vi "Sect02-Single File_Write Results.vi"(8 "error in (no error)":errorcluster, 11 "QSM_ShiftRegister_TEST in":T1 {"ROI Process"."Particle Variables" items=["Center of Mass X", "Center of Mass Y", "First Pixel X", "First Pixel Y", "Bounding Rect Left", "Bounding Rect Top", "Bounding Rect Right", "Bounding Rect Bottom", "Max Feret Diameter Start X", "Max Feret Diameter Start Y", "Max Feret Diameter End X", "Max Feret Diameter End Y", "Max Horiz. Segment Length Left", "Max Horiz. Segment Length Right", "Max Horiz. Segment Length Row", "-", "Bounding Rect Width", "Bounding Rect Height", "Bounding Rect Diagonal", "Perimeter", "Convex Hull Perimeter", "Holes' Perimeter", "Max Feret Diameter", "Equivalent Ellipse Major Axis", "Equivalent Ellipse Minor Axis", "Equivalent Ellipse Minor Axis (Feret)", "Equivalent Rect Long Side", "Equivalent Rect Short Side", "Equivalent Rect Diagonal", "Equivalent Rect Short Side (Feret)", "Average Horiz. Segment Length", "Average Vert. Segment Length", "Hydraulic Radius", "Waddel Disk Diameter", "-", "Area", "Holes' Area", "Particle & Holes' Area", "Convex Hull Area", "Image Area", "-", "Number of Holes", "Number of Horiz. Segments", "Number of Vert. Segments", "-", "Orientation", "Max Feret Diameter Orientation", "-", "% Area/Image Area", "% Area/(Particle & Holes' Area)", "Ratio of Equivalent Ellipse Axes", "Ratio of Equivalent Rect Sides", "-", "Elongation Factor", "Compactness Factor", "Heywood Circularity Factor", "Type Factor", "-", "Sum X", "Sum Y", "Sum XX", "Sum XY", "Sum YY", "Sum XXX", "Sum XXY", "Sum XYY", "Sum YYY", "-", "Moment of Inertia XX", "Moment of Inertia XY", "Moment of Inertia YY", "Moment of Inertia XXX", "Moment of Inertia XXY", "Moment of Inertia XYY", "Moment of Inertia YYY", "Norm. Moment of Inertia XX", "Norm. Moment of Inertia XY", "Norm. Moment of Inertia YY", "Norm. Moment of Inertia XXX", "Norm. Moment of Inertia XXY", "Norm. Moment of Inertia XYY", "Norm. Moment of Inertia YYY", "Hu Moment 1", "Hu Moment 2", "Hu Moment 3", "Hu Moment 4", "Hu Moment 5", "Hu Moment 6", "Hu Moment 7"]; "ROI Process"."Particle Measurements (Pixels)" format="%.2f"; "ROI Process"."ROIS"."Contours"."Type" items=["No Selection", "Point", "Line", "Rectangle", "Oval", "Polygon", "Freehand Region", "Annulus", "Unused2", "Unused3", "Broken Line", "Freehand Line", "Rotated Rectangle"]; "Single Image Results"."ROI Results"."LIMLOCALMETADATA"."dTimeMSec" format="%.2f"}) -> (0 "error out":errorcluster, 3 "QSM_ShiftRegister_TEST out":T1 {"ROI Process"."Particle Variables" items=["Center of Mass X", "Center of Mass Y", "First Pixel X", "First Pixel Y", "Bounding Rect Left", "Bounding Rect Top", "Bounding Rect Right", "Bounding Rect Bottom", "Max Feret Diameter Start X", "Max Feret Diameter Start Y", "Max Feret Diameter End X", "Max Feret Diameter End Y", "Max Horiz. Segment Length Left", "Max Horiz. Segment Length Right", "Max Horiz. Segment Length Row", "-", "Bounding Rect Width", "Bounding Rect Height", "Bounding Rect Diagonal", "Perimeter", "Convex Hull Perimeter", "Holes' Perimeter", "Max Feret Diameter", "Equivalent Ellipse Major Axis", "Equivalent Ellipse Minor Axis", "Equivalent Ellipse Minor Axis (Feret)", "Equivalent Rect Long Side", "Equivalent Rect Short Side", "Equivalent Rect Diagonal", "Equivalent Rect Short Side (Feret)", "Average Horiz. Segment Length", "Average Vert. Segment Length", "Hydraulic Radius", "Waddel Disk Diameter", "-", "Area", "Holes' Area", "Particle & Holes' Area", "Convex Hull Area", "Image Area", "-", "Number of Holes", "Number of Horiz. Segments", "Number of Vert. Segments", "-", "Orientation", "Max Feret Diameter Orientation", "-", "% Area/Image Area", "% Area/(Particle & Holes' Area)", "Ratio of Equivalent Ellipse Axes", "Ratio of Equivalent Rect Sides", "-", "Elongation Factor", "Compactness Factor", "Heywood Circularity Factor", "Type Factor", "-", "Sum X", "Sum Y", "Sum XX", "Sum XY", "Sum YY", "Sum XXX", "Sum XXY", "Sum XYY", "Sum YYY", "-", "Moment of Inertia XX", "Moment of Inertia XY", "Moment of Inertia YY", "Moment of Inertia XXX", "Moment of Inertia XXY", "Moment of Inertia XYY", "Moment of Inertia YYY", "Norm. Moment of Inertia XX", "Norm. Moment of Inertia XY", "Norm. Moment of Inertia YY", "Norm. Moment of Inertia XXX", "Norm. Moment of Inertia XXY", "Norm. Moment of Inertia XYY", "Norm. Moment of Inertia YYY", "Hu Moment 1", "Hu Moment 2", "Hu Moment 3", "Hu Moment 4", "Hu Moment 5", "Hu Moment 6", "Hu Moment 7"]; "ROI Process"."Particle Measurements (Pixels)" format="%.2f"; "ROI Process"."ROIS"."Contours"."Type" items=["No Selection", "Point", "Line", "Rectangle", "Oval", "Polygon", "Freehand Region", "Annulus", "Unused2", "Unused3", "Broken Line", "Freehand Line", "Rotated Rectangle"]; "Single Image Results"."ROI Results"."LIMLOCALMETADATA"."dTimeMSec" format="%.2f"})   [LabVIEW 2014, in "TestQSM.lvlib"]
uses:
  TestQSM.lvlib
  Controls/QSM_ShiftRegister.ctl
  QueueMaintenance/TypeDef/QSMRef_ALL.ctl
  Queue_TESTGUIUPDATE/Controls/QSM_Reference.ctl
  Queue_TESTGUIUPDATE/Controls/QSM_DataType.ctl
  Queue_TESTGUIUPDATE/Controls/QSM_RunStates.ctl
  Controls/QSM_Reference.ctl
  Controls/QSM_DataType.ctl
  Controls/QSM_RunStates.ctl
  Custom Controls/cluster - Image Results.ctl
  ND2_Reader_32bit/controls/cluster_LIMLOCALMETADATA.ctl
  FileIO/TypeDef - File Actions.ctl
  Queue_TESTGUIUPDATE/GUIUpdateQSM.lvlib
  QueueMaintenance/QueueMaintenance.lvlib
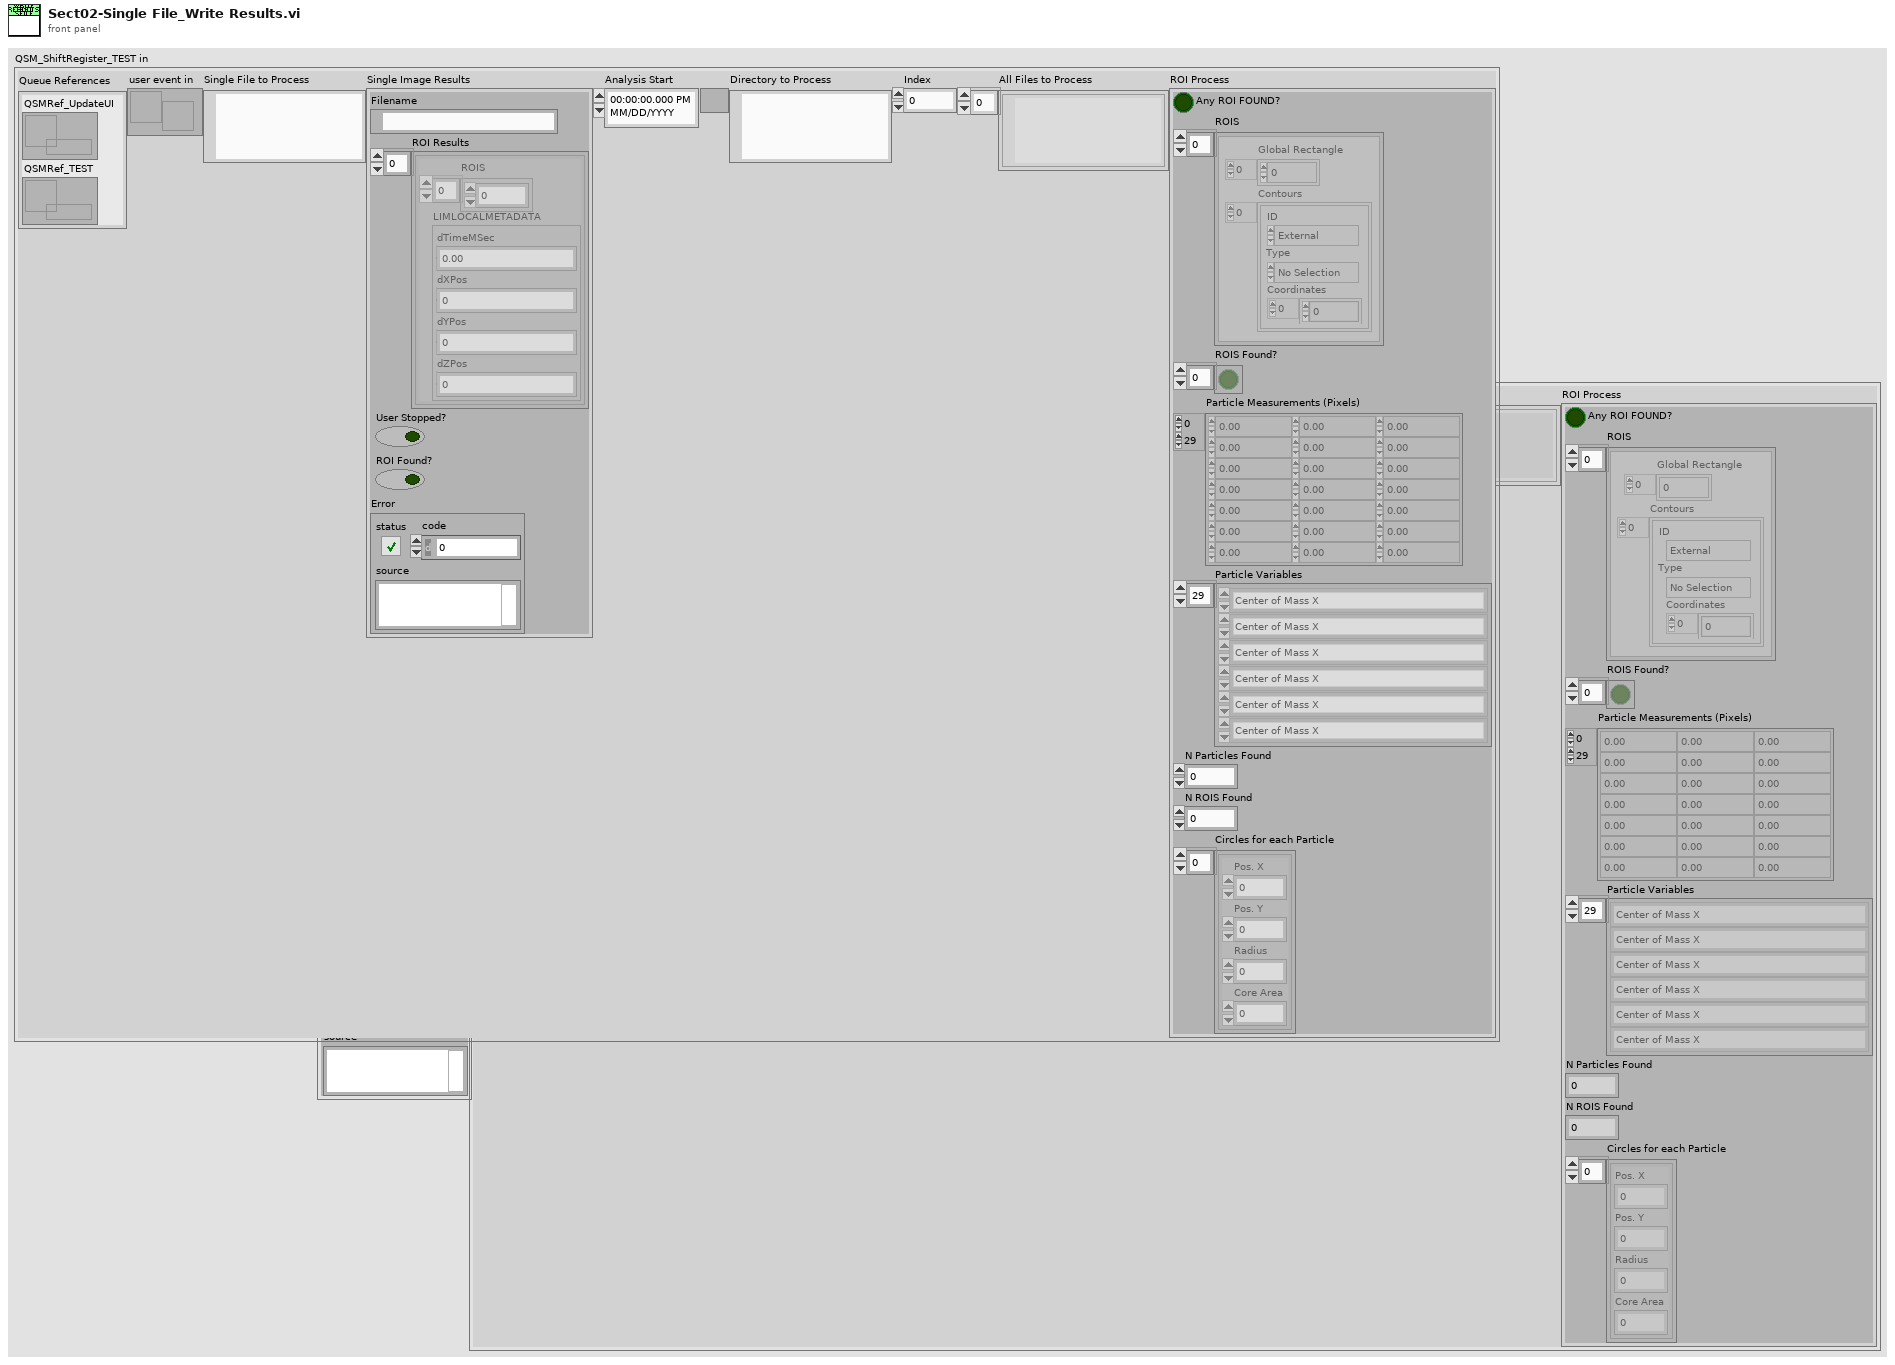
[diagram p1: front panel]
types:
  T1 = typedef "TestQSM.lvlib/QSM_ShiftRegister.ctl" = cluster{"Queue References":T2, "user event in":refnum<user-event>, "Single File to Process":path, "Single Image Results":T5, "Analysis Start":timestamp, "Directory to Process":path, "Index":i32, "All Files to Process":path[], "ROI Process":cluster{"Any ROI FOUND?":bool, "ROIS":T7[], "ROIS Found?":bool[], "Particle Measurements (Pixels)":dbl[][], "Particle Variables":i32[], "N Particles Found":i32, "N ROIS Found":i32, "Circles for each Particle":cluster{"Pos. X":i32, "Pos. Y":i32, "Radius":i32, "Core Area":i32}[]}}
  T2 = typedef "QueueMaintenance.lvlib/QSMRef_ALL.ctl" = cluster{"QSMRef_UpdateUI":T3, "QSMRef_TEST":T4}
  T3 = typedef "GUIUpdateQSM.lvlib/QSM_Reference.ctl" = refnum<queue>
  T4 = typedef "TestQSM.lvlib/QSM_Reference.ctl" = refnum<queue>
  T5 = typedef "cluster - Image Results.ctl" = cluster{"Filename":path, "ROI Results":cluster{"ROIS":dbl[], "LIMLOCALMETADATA":T6}[], "User Stopped?":bool, "ROI Found?":bool, "Error":errorcluster}
  T6 = typedef "cluster_LIMLOCALMETADATA.ctl" = cluster{"dTimeMSec":dbl, "dXPos":dbl, "dYPos":dbl, "dZPos":dbl}
  T7 = typedef "ROI Descriptor" = cluster{"Global Rectangle":i32[], "Contours":cluster{"ID":enum32{"External", "Internal"}, "Type":u32, "Coordinates":i32[]}[]}
  T8 = typedef "TypeDef - File Actions.ctl" = enum16{"Read", "Write", "Get Current"}
  T9 = cluster{"Any ROI FOUND?":bool, "ROIS":T7[], "ROIS Found?":bool[], "Particle Measurements (Pixels)":dbl[][], "Particle Variables":i32[], "N Particles Found":i32, "N ROIS Found":i32, "Circles for each Particle":cluster{"Pos. X":i32, "Pos. Y":i32, "Radius":i32, "Core Area":i32}[]}
  T10 = typedef "TypeDef - System Configuration.ctl" = cluster{"Results FilePath":path, "Analysis Parameters":cluster{"Area":cluster{"Lower Value":dbl, "Upper Value":dbl}, "Circle Filter Radius":cluster{"Lower Value":sgl, "Upper Value":sgl}, "Edge Detection Threshold":u16}, "ROI Parameters":cluster{"ROI size (in Radius)":cluster{"Width":dbl, "Height":dbl}}}
  T11 = enum16{"open", "replace", "create", "open or create", "replace or create", "replace or create with confirmation"}
  T12 = cluster{"Pos. X":i32, "Pos. Y":i32, "Radius":i32, "Core Area":i32}[]
  T13 = cluster{"Pos. X":i32, "Pos. Y":i32, "Radius":i32, "Core Area":i32}
  T14 = cluster{"Pos. X":string, "Pos. Y":string, "Radius":string, "Core Area":string}
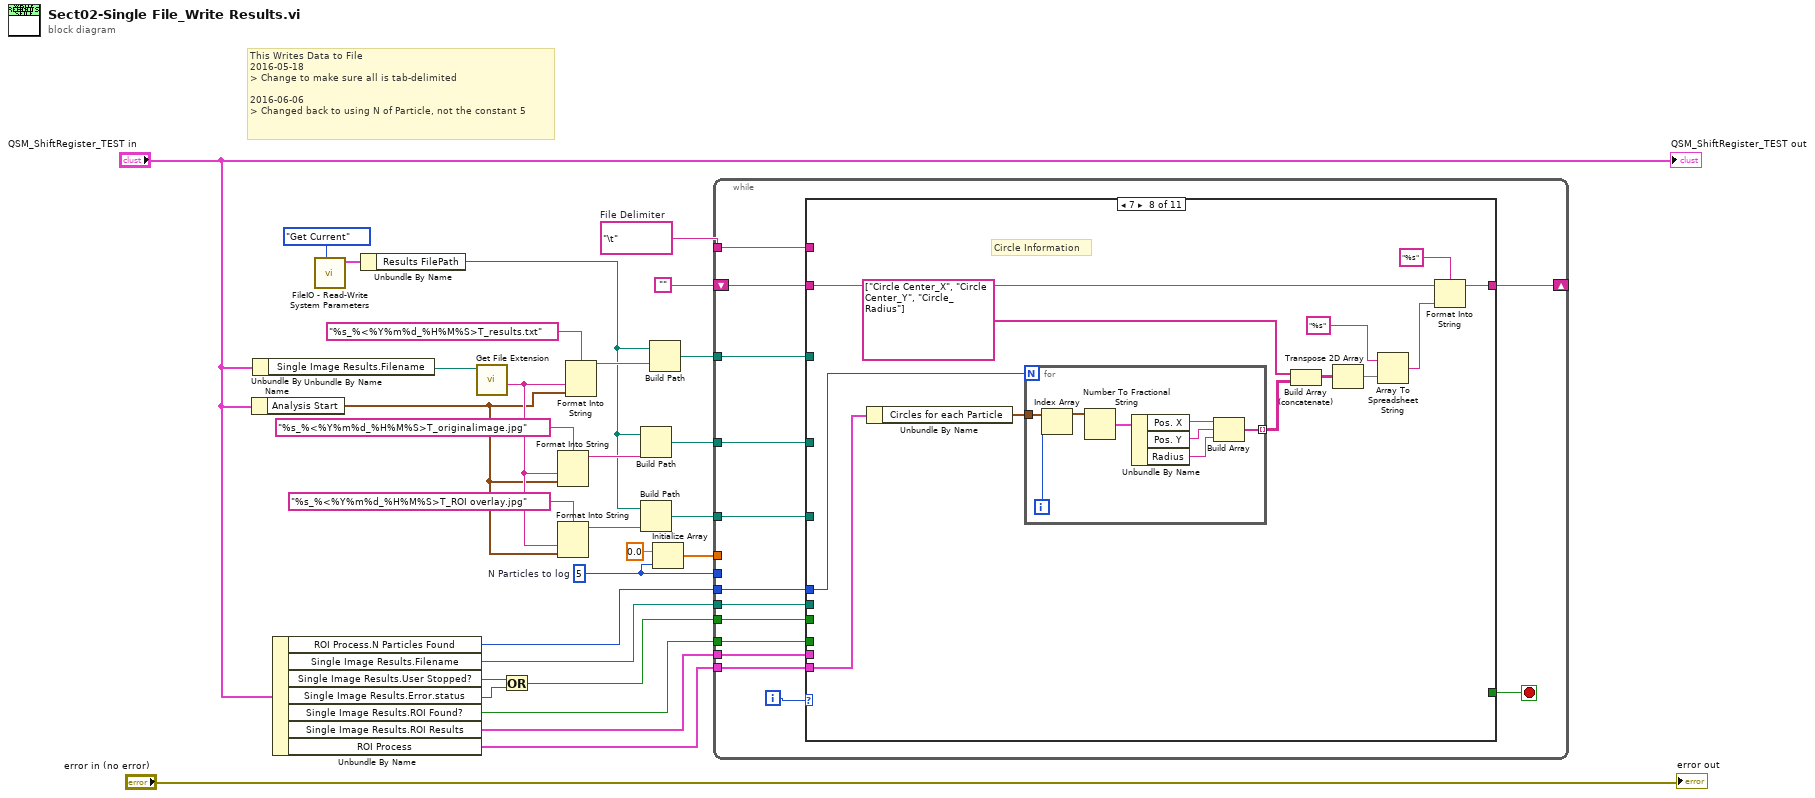
[diagram p0: block diagram]
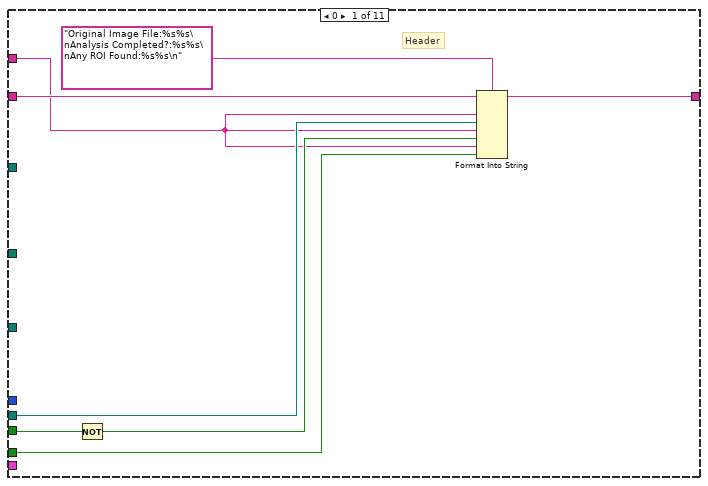
[diagram p2: hidden frame]
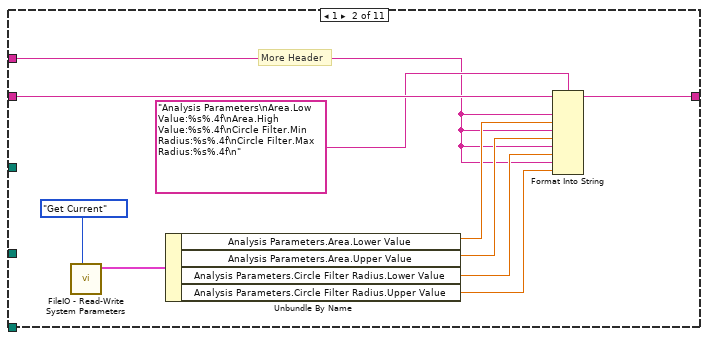
[diagram p3: hidden frame]
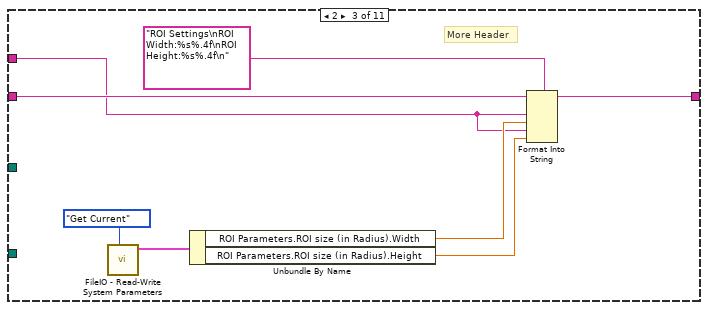
[diagram p4: hidden frame]
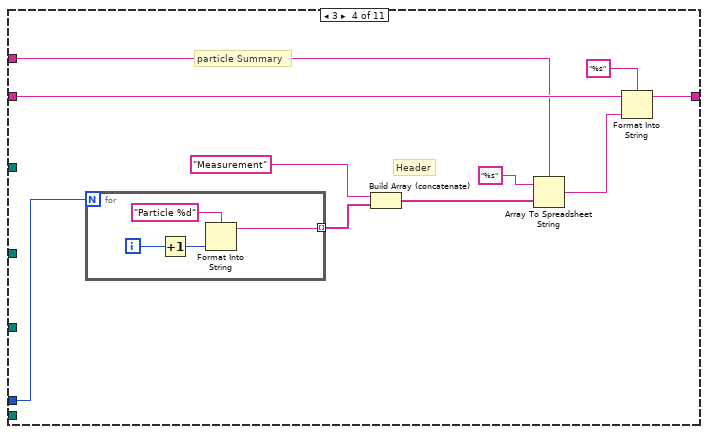
[diagram p5: hidden frame]
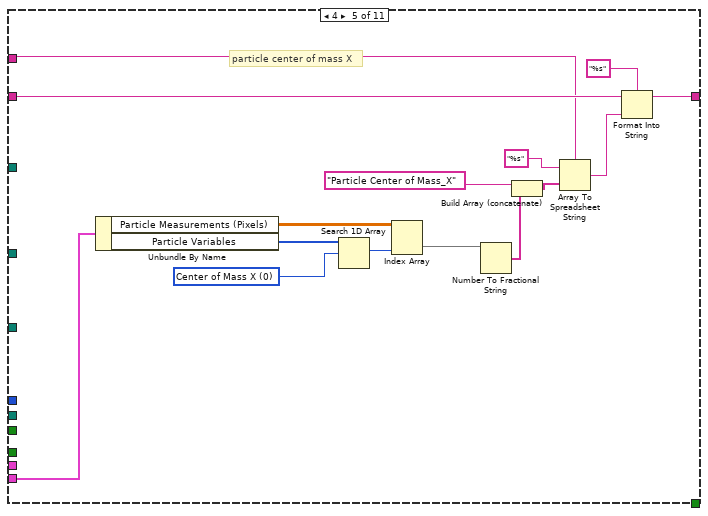
[diagram p6: hidden frame]
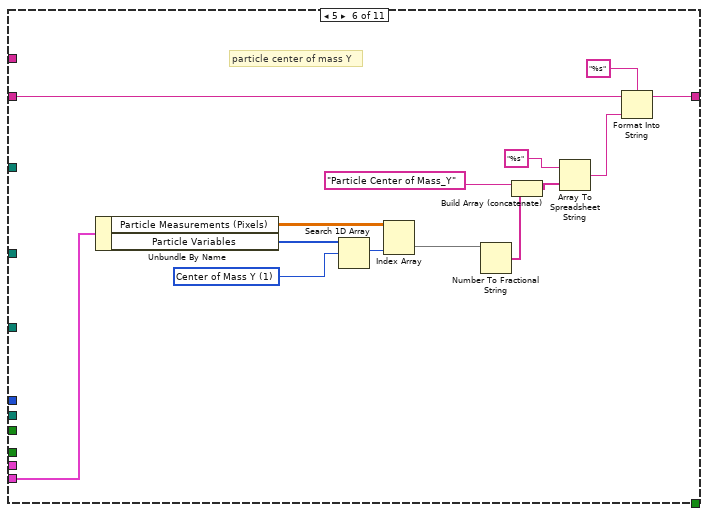
[diagram p7: hidden frame]
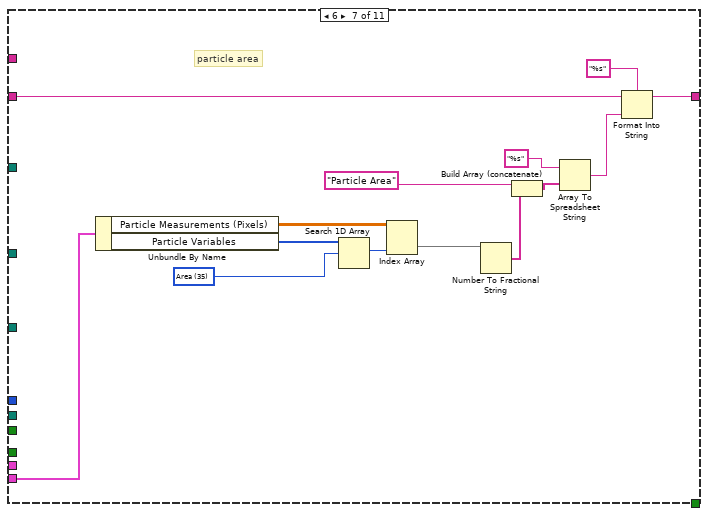
[diagram p8: hidden frame]
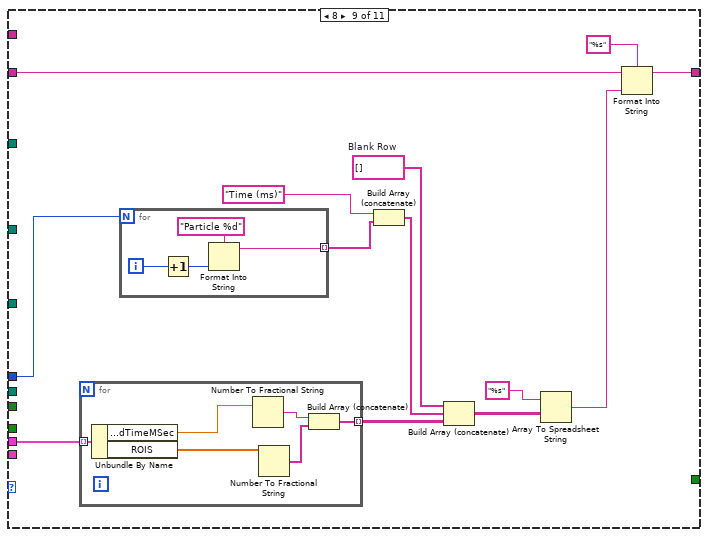
[diagram p9: hidden frame]
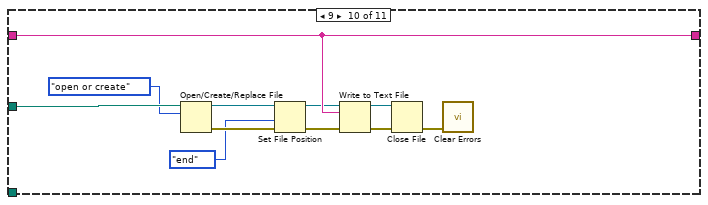
[diagram p10: hidden frame]
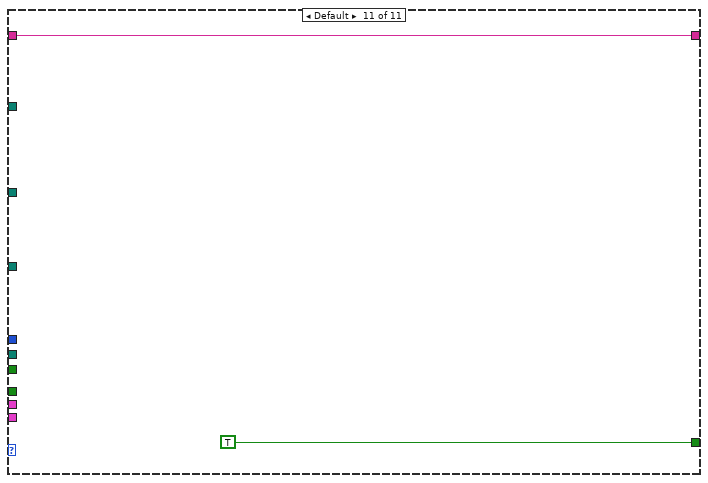
[diagram p11: hidden frame]
diagram:
  w4 = "\t"  # File Delimiter
  w3 = 5  # N Particles to log
  # "This Writes Data to File\n2016-05-18\n> Change to make sure all is tab-delimited\n\n2016-06-06\n> Changed back to using N of Particle, not the constant 5"
  n1 = Unbundle By Name("QSM_ShiftRegister_TEST in") -> ("Analysis Start"=w9:timestamp)
  n2 = Unbundle By Name("QSM_ShiftRegister_TEST in") -> ("Single Image Results.Filename"=w29:path)
  n3 = Unbundle By Name("QSM_ShiftRegister_TEST in") -> ("ROI Process.N Particles Found"=w6:i32, "Single Image Results.Filename"=w22:path, "Single Image Results.User Stopped?"=w18:bool, "Single Image Results.Error.status"=w17:bool, "Single Image Results.ROI Found?"=w21:bool, "Single Image Results.ROI Results"=w19:cluster{"ROIS":dbl[], "LIMLOCALMETADATA":T6}[], "ROI Process"=w5:T9)
  n4 = call "FileIO - Read-Write System Parameters.vi"("Action"=TypeDef_-_File_Actions."Get Current") -> ("System Parameters out"=w25:T10)  [unwired: 9 in, 1 out]
  n5 = Unbundle By Name(w25) -> ("Results FilePath"=w8:path)
  n6 = call <vilib>:"Get File Extension.vi"("file"=w29) -> ("filename without extension"=w10:string)  [unwired: 7 in, 3 out]
  n7 = Or(x=w18, y=w17) -> (x .or. y?=w16:bool)
  n8 = Format Into String(format string="%s_%<%Y%m%d_%H%M%S>T_originalimage.jpg", w10, w9) -> (resulting string=w14:string)  [unwired: 2 in, 1 out]
  n9 = Format Into String(format string="%s_%<%Y%m%d_%H%M%S>T_ROI overlay.jpg", w10, w9) -> (resulting string=w12:string)  [unwired: 2 in, 1 out]
  n10 = Format Into String(format string="%s_%<%Y%m%d_%H%M%S>T_results.txt", w10, w9) -> (resulting string=w26:string)  [unwired: 2 in, 1 out]
  n11 = Build Path(base path=w8, name or relative path=w14) -> (appended path=w13:path)
  n12 = Build Path(base path=w8, name or relative path=w12) -> (appended path=w7:path)
  n13 = Build Path(base path=w8, name or relative path=w26) -> (appended path=w24:path)
  n14 = Initialize Array(0.0 ("element"), w3) -> (w1:dbl[])
  n15 = while {
    tunnel: w24 -> [w42]
    shift-right: [w41] -> _
    shift-left: "" -> [w40]
    tunnel: w16 -> [w39]
    tunnel: w22 -> [w38]
    tunnel: w21 -> [w37]
    tunnel: w19 -> [w36]
    tunnel: w13 -> [w35]
    tunnel: w7 -> [w34]
    tunnel: w6 -> [w31]
    tunnel: w5 -> [w33]
    tunnel: w3 -> [_]
    tunnel: w4 -> [w32]
    tunnel: w1 -> [_]
    i -> [w44]
    stop <- w43 stop-if-true
    n16 = case shown="7" w44 {
      tunnel: [_ _ _ _ _ _ _ _ _ _ TRUE] -> w43
      tunnel: w42 -> [_ _ _ _ _ _ _ _ _ w173 _]
      tunnel: [w51 w58 w66 w79 w98 w112 w126 w138 w159 w178 w182] -> w41
      tunnel: w40 -> [w52 w60 w68 w80 w99 w113 w127 w139 w160 w178 w182]
      tunnel: w39 -> [w50 _ _ _ _ _ _ _ _ _ _]
      tunnel: w38 -> [w46 _ _ _ _ _ _ _ _ _ _]
      tunnel: w37 -> [w48 _ _ _ _ _ _ _ _ _ _]
      tunnel: w36 -> [_ _ _ _ _ _ _ _ w151 _ _]
      tunnel: w35 -> [_ _ _ _ _ _ _ _ _ _ _]
      tunnel: w34 -> [_ _ _ _ _ _ _ _ _ _ _]
      tunnel: w31 -> [_ _ _ w71 _ _ _ w128 w148 _ _]
      tunnel: w33 -> [_ _ _ _ w96 w110 w124 w136 _ _ _]
      tunnel: w32 -> [w45 w53 w63 w72 w86 _ _ _ _ _ _]
      frame 0 {
        # "Header"
        n17 = Not(x=w50) -> (.not. x?=w49:bool)
        n18 = Format Into String(format string="Original Image File:%s%s\nAnalysis Completed?:%s%s\nAny ROI Found:%s%s\n", initial string=w52, w45, w46, w45, w49, w45, w48) -> (resulting string=w51:string)  [unwired: 1 in, 1 out]
      }
      frame 1 {
        # "More Header"
        n19 = call "FileIO - Read-Write System Parameters.vi"("Action"=TypeDef_-_File_Actions."Get Current") -> ("System Parameters out"=w61:T10)  [unwired: 9 in, 1 out]
        n20 = Unbundle By Name(w61) -> ("Analysis Parameters.Area.Lower Value"=w57:dbl, "Analysis Parameters.Area.Upper Value"=w56:dbl, "Analysis Parameters.Circle Filter Radius.Lower Value"=w55:sgl, "Analysis Parameters.Circle Filter Radius.Upper Value"=w54:sgl)
        n21 = Format Into String(format string="Analysis Parameters\nArea.Low Value:%s%.4f\nArea.High Value:%s%.4f\nCircle Filter.Min Radius:%s%.4f\nCircle Filter.Max Radius:%s%.4f\n", initial string=w60, w53, w57, w53, w56, w53, w55, w53, w54) -> (resulting string=w58:string)  [unwired: 1 in, 1 out]
      }
      frame 2 {
        # "More Header"
        n22 = call "FileIO - Read-Write System Parameters.vi"("Action"=TypeDef_-_File_Actions."Get Current") -> ("System Parameters out"=w69:T10)  [unwired: 9 in, 1 out]
        n23 = Unbundle By Name(w69) -> ("ROI Parameters.ROI size (in Radius).Width"=w65:dbl, "ROI Parameters.ROI size (in Radius).Height"=w64:dbl)
        n24 = Format Into String(format string="ROI Settings\nROI Width:%s%.4f\nROI Height:%s%.4f\n", initial string=w68, w63, w65, w63, w64) -> (resulting string=w66:string)  [unwired: 1 in, 1 out]
      }
      frame 3 {
        # "Header"
        # "particle Summary"
        n25 = for {
          N: w71 -> [_]
          tunnel: [w82] -> w74 mode=indexing
          i -> [w81]
          n26 = Increment(x=w81) -> (x+1=w83:i32)
          n27 = Format Into String(format string="Particle %d", w83) -> (resulting string=w82:string)  [unwired: 2 in, 1 out]
        }
        n28 = Build Array (concatenate)("Measurement" ("format string"), w74) -> (w73:string[])
        n29 = Array To Spreadsheet String(delimiter (Tab)=w72, array=w73, 3:"%s" ("format string")) -> (spreadsheet string=w75:string)
        n30 = Format Into String(format string="%s", initial string=w80, w75) -> (resulting string=w79:string)  [unwired: 1 in, 1 out]
      }
      frame 4 {
        w94 = 0 items=["Center of Mass X", "Center of Mass Y", "First Pixel X", "First Pixel Y", "Bounding Rect Left", "Bounding Rect Top", "Bounding Rect Right", "Bounding Rect Bottom", "Max Feret Diameter Start X", "Max Feret Diameter Start Y", "Max Feret Diameter End X", "Max Feret Diameter End Y", "Max Horiz. Segment Length Left", "Max Horiz. Segment Length Right", "Max Horiz. Segment Length Row", "-", "Bounding Rect Width", "Bounding Rect Height", "Bounding Rect Diagonal", "Perimeter", "Convex Hull Perimeter", "Holes' Perimeter", "Max Feret Diameter", "Equivalent Ellipse Major Axis", "Equivalent Ellipse Minor Axis", "Equivalent Ellipse Minor Axis (Feret)", "Equivalent Rect Long Side", "Equivalent Rect Short Side", "Equivalent Rect Diagonal", "Equivalent Rect Short Side (Feret)", "Average Horiz. Segment Length", "Average Vert. Segment Length", "Hydraulic Radius", "Waddel Disk Diameter", "-", "Area", "Holes' Area", "Particle & Holes' Area", "Convex Hull Area", "Image Area", "-", "Number of Holes", "Number of Horiz. Segments", "Number of Vert. Segments", "-", "Orientation", "Max Feret Diameter Orientation", "-", "% Area/Image Area", "% Area/(Particle & Holes' Area)", "Ratio of Equivalent Ellipse Axes", "Ratio of Equivalent Rect Sides", "-", "Elongation Factor", "Compactness Factor", "Heywood Circularity Factor", "Type Factor", "-", "Sum X", "Sum Y", "Sum XX", "Sum XY", "Sum YY", "Sum XXX", "Sum XXY", "Sum XYY", "Sum YYY", "-", "Moment of Inertia XX", "Moment of Inertia XY", "Moment of Inertia YY", "Moment of Inertia XXX", "Moment of Inertia XXY", "Moment of Inertia XYY", "Moment of Inertia YYY", "Norm. Moment of Inertia XX", "Norm. Moment of Inertia XY", "Norm. Moment of Inertia YY", "Norm. Moment of Inertia XXX", "Norm. Moment of Inertia XXY", "Norm. Moment of Inertia XYY", "Norm. Moment of Inertia YYY", "Hu Moment 1", "Hu Moment 2", "Hu Moment 3", "Hu Moment 4", "Hu Moment 5", "Hu Moment 6", "Hu Moment 7"] ("Measurement Parameter")
        # "particle center of mass X"
        n31 = Unbundle By Name(w96) -> ("Particle Measurements (Pixels)"=w93:dbl[][], "Particle Variables"=w95:i32[])
        n32 = Search 1D Array(1D array=w95, element=w94) -> (index of element=w92:i32)  [unwired: 1 in]
        n33 = Index Array(array=w93, index (col)=w92) -> (element=w85:dbl[])  [unwired: 1 in]
        n34 = Number To Fractional String(number=w85) -> (F-format string=w91:string[])  [unwired: 3 in]
        n35 = Build Array (concatenate)("Particle Center of Mass_X" ("Numeric"), w91) -> (w88:string[])
        n36 = Array To Spreadsheet String(delimiter (Tab)=w86, array=w88, 3:"%s" ("format string")) -> (spreadsheet string=w87:string)
        n37 = Format Into String(format string="%s", initial string=w99, w87) -> (resulting string=w98:string)  [unwired: 1 in, 1 out]
      }
      frame 5 {
        w108 = 1 items=["Center of Mass X", "Center of Mass Y", "First Pixel X", "First Pixel Y", "Bounding Rect Left", "Bounding Rect Top", "Bounding Rect Right", "Bounding Rect Bottom", "Max Feret Diameter Start X", "Max Feret Diameter Start Y", "Max Feret Diameter End X", "Max Feret Diameter End Y", "Max Horiz. Segment Length Left", "Max Horiz. Segment Length Right", "Max Horiz. Segment Length Row", "-", "Bounding Rect Width", "Bounding Rect Height", "Bounding Rect Diagonal", "Perimeter", "Convex Hull Perimeter", "Holes' Perimeter", "Max Feret Diameter", "Equivalent Ellipse Major Axis", "Equivalent Ellipse Minor Axis", "Equivalent Ellipse Minor Axis (Feret)", "Equivalent Rect Long Side", "Equivalent Rect Short Side", "Equivalent Rect Diagonal", "Equivalent Rect Short Side (Feret)", "Average Horiz. Segment Length", "Average Vert. Segment Length", "Hydraulic Radius", "Waddel Disk Diameter", "-", "Area", "Holes' Area", "Particle & Holes' Area", "Convex Hull Area", "Image Area", "-", "Number of Holes", "Number of Horiz. Segments", "Number of Vert. Segments", "-", "Orientation", "Max Feret Diameter Orientation", "-", "% Area/Image Area", "% Area/(Particle & Holes' Area)", "Ratio of Equivalent Ellipse Axes", "Ratio of Equivalent Rect Sides", "-", "Elongation Factor", "Compactness Factor", "Heywood Circularity Factor", "Type Factor", "-", "Sum X", "Sum Y", "Sum XX", "Sum XY", "Sum YY", "Sum XXX", "Sum XXY", "Sum XYY", "Sum YYY", "-", "Moment of Inertia XX", "Moment of Inertia XY", "Moment of Inertia YY", "Moment of Inertia XXX", "Moment of Inertia XXY", "Moment of Inertia XYY", "Moment of Inertia YYY", "Norm. Moment of Inertia XX", "Norm. Moment of Inertia XY", "Norm. Moment of Inertia YY", "Norm. Moment of Inertia XXX", "Norm. Moment of Inertia XXY", "Norm. Moment of Inertia XYY", "Norm. Moment of Inertia YYY", "Hu Moment 1", "Hu Moment 2", "Hu Moment 3", "Hu Moment 4", "Hu Moment 5", "Hu Moment 6", "Hu Moment 7"] ("Measurement Parameter")
        # "particle center of mass Y"
        n38 = Unbundle By Name(w110) -> ("Particle Measurements (Pixels)"=w107:dbl[][], "Particle Variables"=w109:i32[])
        n39 = Search 1D Array(1D array=w109, element=w108) -> (index of element=w106:i32)  [unwired: 1 in]
        n40 = Index Array(array=w107, index (col)=w106) -> (element=w100:dbl[])  [unwired: 1 in]
        n41 = Number To Fractional String(number=w100) -> (F-format string=w105:string[])  [unwired: 3 in]
        n42 = Build Array (concatenate)("Particle Center of Mass_Y" ("Numeric"), w105) -> (w102:string[])
        n43 = Array To Spreadsheet String(array=w102, 3:"%s" ("format string")) -> (spreadsheet string=w101:string)  [unwired: 1 in]
        n44 = Format Into String(format string="%s", initial string=w113, w101) -> (resulting string=w112:string)  [unwired: 1 in, 1 out]
      }
      frame 6 {
        w122 = 35 items=["Center of Mass X", "Center of Mass Y", "First Pixel X", "First Pixel Y", "Bounding Rect Left", "Bounding Rect Top", "Bounding Rect Right", "Bounding Rect Bottom", "Max Feret Diameter Start X", "Max Feret Diameter Start Y", "Max Feret Diameter End X", "Max Feret Diameter End Y", "Max Horiz. Segment Length Left", "Max Horiz. Segment Length Right", "Max Horiz. Segment Length Row", "-", "Bounding Rect Width", "Bounding Rect Height", "Bounding Rect Diagonal", "Perimeter", "Convex Hull Perimeter", "Holes' Perimeter", "Max Feret Diameter", "Equivalent Ellipse Major Axis", "Equivalent Ellipse Minor Axis", "Equivalent Ellipse Minor Axis (Feret)", "Equivalent Rect Long Side", "Equivalent Rect Short Side", "Equivalent Rect Diagonal", "Equivalent Rect Short Side (Feret)", "Average Horiz. Segment Length", "Average Vert. Segment Length", "Hydraulic Radius", "Waddel Disk Diameter", "-", "Area", "Holes' Area", "Particle & Holes' Area", "Convex Hull Area", "Image Area", "-", "Number of Holes", "Number of Horiz. Segments", "Number of Vert. Segments", "-", "Orientation", "Max Feret Diameter Orientation", "-", "% Area/Image Area", "% Area/(Particle & Holes' Area)", "Ratio of Equivalent Ellipse Axes", "Ratio of Equivalent Rect Sides", "-", "Elongation Factor", "Compactness Factor", "Heywood Circularity Factor", "Type Factor", "-", "Sum X", "Sum Y", "Sum XX", "Sum XY", "Sum YY", "Sum XXX", "Sum XXY", "Sum XYY", "Sum YYY", "-", "Moment of Inertia XX", "Moment of Inertia XY", "Moment of Inertia YY", "Moment of Inertia XXX", "Moment of Inertia XXY", "Moment of Inertia XYY", "Moment of Inertia YYY", "Norm. Moment of Inertia XX", "Norm. Moment of Inertia XY", "Norm. Moment of Inertia YY", "Norm. Moment of Inertia XXX", "Norm. Moment of Inertia XXY", "Norm. Moment of Inertia XYY", "Norm. Moment of Inertia YYY", "Hu Moment 1", "Hu Moment 2", "Hu Moment 3", "Hu Moment 4", "Hu Moment 5", "Hu Moment 6", "Hu Moment 7"] ("Measurement Parameter")
        # "particle area"
        n45 = Unbundle By Name(w124) -> ("Particle Measurements (Pixels)"=w121:dbl[][], "Particle Variables"=w123:i32[])
        n46 = Search 1D Array(1D array=w123, element=w122) -> (index of element=w120:i32)  [unwired: 1 in]
        n47 = Index Array(array=w121, index (col)=w120) -> (element=w114:dbl[])  [unwired: 1 in]
        n48 = Number To Fractional String(number=w114) -> (F-format string=w119:string[])  [unwired: 3 in]
        n49 = Build Array (concatenate)("Particle Area" ("Numeric"), w119) -> (w116:string[])
        n50 = Array To Spreadsheet String(array=w116, 3:"%s" ("format string")) -> (spreadsheet string=w115:string)  [unwired: 1 in]
        n51 = Format Into String(format string="%s", initial string=w127, w115) -> (resulting string=w126:string)  [unwired: 1 in, 1 out]
      }
      frame 7 {
        # "Circle Information"
        n52 = Unbundle By Name(w136) -> ("Circles for each Particle"=w133:T12)
        n53 = for {
          N: w128 -> [_]
          tunnel: w133 -> [w142]
          tunnel: [w143] -> w129 mode=indexing
          i -> [w140]
          n54 = Index Array(array=w142, index=w140) -> (element=w141:T13)
          n55 = Number To Fractional String(number=w141) -> (F-format string=w147:T14)  [unwired: 3 in]
          n56 = Unbundle By Name(w147) -> ("Pos. X"=w146:string, "Pos. Y"=w145:string, "Radius"=w144:string)
          n57 = Build Array(w146, w145, w144) -> (w143:string[])
        }
        n58 = Build Array (concatenate)(string[] ["Circle Center_X", "Circle Center_Y", "Circle_Radius"], w129) -> (w131:string[][])
        n59 = Transpose 2D Array(2D array=w131) -> (transposed array=w130:string[][])
        n60 = Array To Spreadsheet String(array=w130, 3:"%s" ("format string")) -> (spreadsheet string=w134:string)  [unwired: 1 in]
        n61 = Format Into String(format string="%s", initial string=w139, w134) -> (resulting string=w138:string)  [unwired: 1 in, 1 out]
      }
      frame 8 {
        w149 = string[] []  # Blank Row
        n62 = for {
          tunnel: w151 -> [w170] mode=indexing
          tunnel: [w166] -> w153 mode=indexing
          n63 = Unbundle By Name(w170) -> ("LIMLOCALMETADATA.dTimeMSec"=w169:dbl, "ROIS"=w165:dbl[])
          n64 = Number To Fractional String(number=w169) -> (F-format string=w168:string)  [unwired: 3 in]
          n65 = Number To Fractional String(number=w165) -> (F-format string=w167:string[])  [unwired: 3 in]
          n66 = Build Array (concatenate)(w168, w167) -> (w166:string[])
        }
        n67 = for {
          N: w148 -> [_]
          tunnel: [w162] -> w150 mode=indexing
          i -> [w161]
          n68 = Increment(x=w161) -> (x+1=w163:i32)
          n69 = Format Into String(format string="Particle %d", w163) -> (resulting string=w162:string)  [unwired: 2 in, 1 out]
        }
        n70 = Build Array (concatenate)("Time (ms)" ("format string"), w150) -> (w152:string[])
        n71 = Build Array (concatenate)(w149, w152, w153) -> (w154:string[][])
        n72 = Array To Spreadsheet String(array=w154, 3:"%s" ("format string")) -> (spreadsheet string=w155:string)  [unwired: 1 in]
        n73 = Format Into String(format string="%s", initial string=w160, w155) -> (resulting string=w159:string)  [unwired: 1 in, 1 out]
      }
      frame 9 {
        n74 = Open/Create/Replace File(file path (use dialog)=w173, operation (0:open)=T11."open or create") -> (refnum out=w175:refnum<file>, error out=w174:errorcluster)  [unwired: 4 in, 1 out]
        n75 = Set File Position(refnum=w175, from (0:start)=enum16{"start", "end", "current"}."end", error in=w174) -> (refnum out=w177:refnum<file>, error out=w176:errorcluster)  [unwired: 1 in]
        n76 = Write to Text File(file (use dialog)=w177, text=w178, error in=w176) -> (refnum out=w181:refnum<file>, error out=w180:errorcluster)  [unwired: 1 in, 1 out]
        n77 = Close File(refnum=w181, error in=w180) -> (error out=w179:errorcluster)  [unwired: 1 out]
        n78 = call <vilib>:"Clear Errors.vi"("error in (no error)"=w179) -> ()  [unwired: 5 in, 2 out]
      }
      frame Default {
      }
    }
  }
  "error out" <- "error in (no error)"
  "QSM_ShiftRegister_TEST out" <- "QSM_ShiftRegister_TEST in"
